vi "obtain_instance_queue.vi"(8 "error in (no error)":errorcluster, 11 "GenericToplevelComponent in":refnum<class "GenericToplevelComponent.lvclass">) -> (0 "error out":errorcluster, 2 "instance queue":refnum<queue>, 3 "GenericToplevelComponent out":refnum<class "GenericToplevelComponent.lvclass">)   [LabVIEW 2010, in "GenericToplevelComponent.lvclass"]
uses:
  GenericToplevelComponent.lvclass
  GenericComponent/GenericComponent/GenericComponent.lvclass
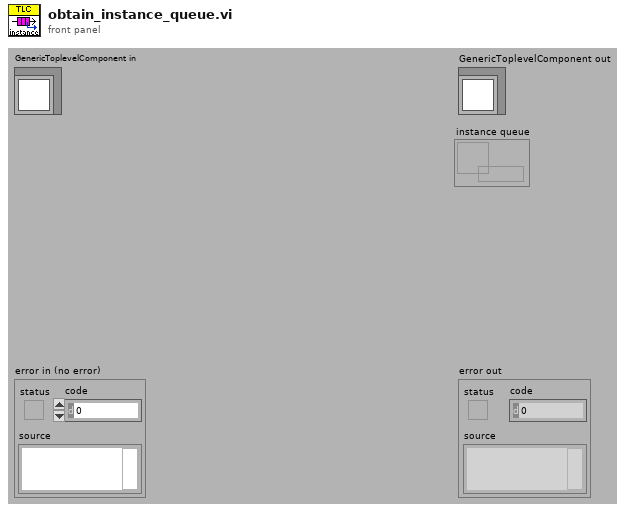
[diagram p1: front panel]
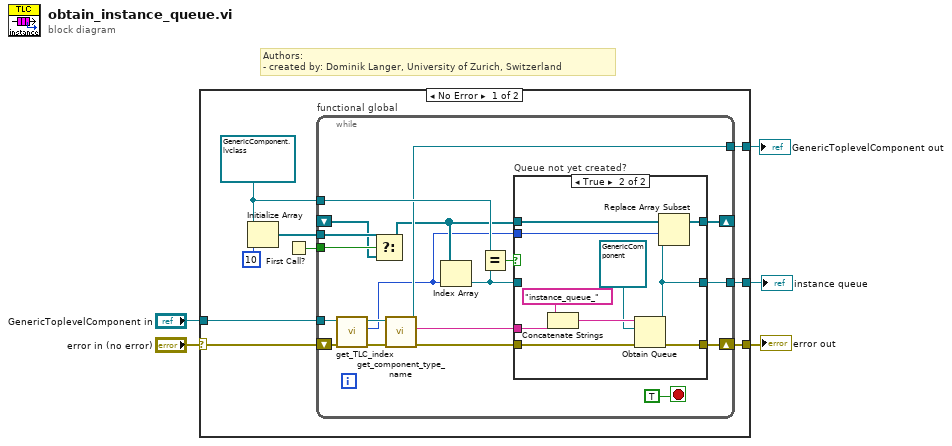
[diagram p0: block diagram]
diagram:
  # "Authors: \n- created by: Dominik Langer, University of Zurich, Switzerland"
  n1 = case shown="No Error" "error in (no error)" {
    selector: "error in (no error)" -> [w9 w48]
    tunnel: [w13 w47] -> w1
    tunnel: "GenericToplevelComponent in" -> [w12 w47]
    tunnel: [w11 _] -> w2
    tunnel: [w10 w48] -> w3
    frame No Error {
      w6 = refnum<queue> refnum ("x")
      n2 = Initialize Array(w6, 10 ("dimension size")) -> (w8:refnum<queue>[])
      n3 = First Call?() -> (First Call?: T/F=w7:bool)
      n4 = while "functional global" {
        shift-right: [w30] -> _
        shift-left: _ -> [w20]
        shift-right: [w29] -> w10
        shift-left: w9 -> [w16]
        tunnel: [w26] -> w11
        tunnel: w6 -> [w25]
        tunnel: [w24] -> w13
        tunnel: w12 -> [w19]
        tunnel: w8 -> [w22]
        tunnel: w7 -> [w23]
        stop <- TRUE stop-if-true
        n5 = call "get_TLC_index.vi"("error in (no error)"=w16, "GenericToplevelComponent in"=w19) -> ("error out"=w15:errorcluster, "index"=w17:i32, "GenericToplevelComponent out"=w18:refnum<class "GenericToplevelComponent.lvclass">)  [unwired: 7 in]
        n6 = Select(t=w22, s=w23, f=w20) -> (s? t:f=w21:refnum<queue>[])
        n7 = call-dynamic "get_component_type_name.vi"("error in (no error)"=w15, "GenericPlugin in"=w18) -> ("error out"=w33:errorcluster, "component type"=w32:string, "GenericPlugin out"=w24:refnum<class "GenericToplevelComponent.lvclass">)  [unwired: 7 in]
        n8 = Index Array(array=w21, index=w17) -> (element=w27:refnum<queue>)
        n9 = Equal?(x=w25, y=w27) -> (x = y?=w31:bool)
        n10 = case "Queue not yet created?" shown="True" w31 {
          tunnel: w33 -> [w36 w45]
          tunnel: w32 -> [_ w44]
          tunnel: [w36 w43] -> w29
          tunnel: w21 -> [w35 w42]
          tunnel: [w35 w39] -> w30
          tunnel: w27 -> [w34 _]
          tunnel: [w34 w40] -> w26
          tunnel: w17 -> [_ w41]
          frame False {
          }
          frame True {
            n11 = Concatenate Strings("instance_queue_" ("string"), w44) -> (w46:string)
            n12 = Obtain Queue(name (unnamed)=w46, element data type=refnum<class "GenericComponent.lvclass"> refnum ("GenericComponent.lvclass"), error in (no error)=w45) -> (queue out=w40:refnum<queue>, error out=w43:errorcluster)  [unwired: 2 in, 1 out]
            n13 = Replace Array Subset(array=w42, new element=w40, index=w41) -> (w39:refnum<queue>[])
          }
        }
      }
    }
    frame Error {
    }
  }
  "error out" <- w3
  "GenericToplevelComponent out" <- w1
  "instance queue" <- w2
